vi "temperaturelimit.vi"() -> ()   [LabVIEW 2022 SP3]
panel:
  out "current":dbl
  out "max":dbl
  out "min":dbl
  in  "Boolean 2":bool
  out "Waveform Chart":T1(graph)
  out "Boolean":bool
  in  "lower limit":dbl
  in  "upper limit":dbl
  # "t"
  # "f"
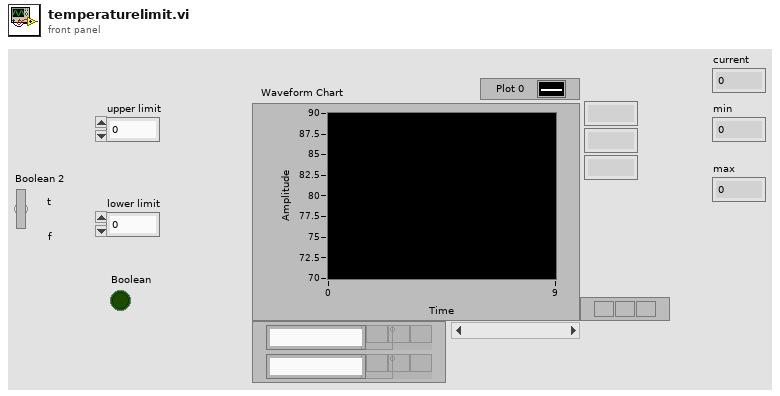
[diagram p1: front panel]
types:
  T1 = cluster{"Thermometer":dbl, "lower limit":dbl, "upper limit":dbl}
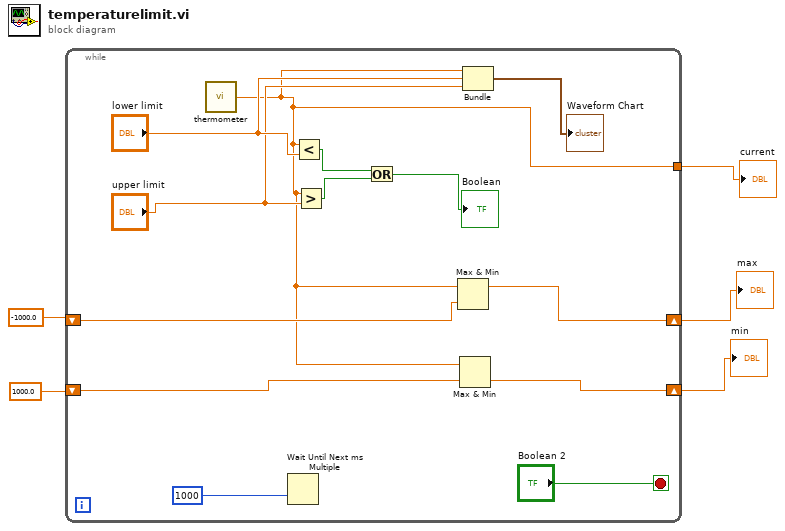
[diagram p0: block diagram]
diagram:
  n1 = while {
    shift-right: [w8] -> w5
    shift-left: -1000.0 -> [w10]
    shift-right: [w7] -> w4
    shift-left: 1000.0 -> [w9]
    tunnel: [w6] -> w3
    stop <- "Boolean 2" stop-if-true
    n2 = call "thermometer.vi"() -> ("Thermometer"=w6:dbl)  [unwired: 1 in]
    n3 = Wait Until Next ms Multiple(millisecond multiple=1000) -> ()  [unwired: 1 out]
    n4 = Less?(x=w6, y="lower limit") -> (x < y?=w18:bool)
    n5 = Greater?(x=w6, y="upper limit") -> (0:w17:bool)
    n6 = Or(x=w18, y=w17) -> (x .or. y?=→"Boolean":bool)
    n7 = Max & Min(x=w6, y=w10) -> (max(x,y)=w8:dbl)  [unwired: 1 out]
    n8 = Max & Min(x=w6, y=w9) -> (min(x,y)=w7:dbl)  [unwired: 1 out]
    n9 = Bundle("Thermometer"=w6, "lower limit"="lower limit", "upper limit"="upper limit") -> (→"Waveform Chart":T1)  [unwired: 1 in]
  }
  "max" <- w5
  "min" <- w4
  "current" <- w3
